vi "TestMirao52e.vi"() -> ()   [LabVIEW 2011]
doc: "This VI is designed to be used with the UDP Receiver VI. Run the UDP Receiver.vi first.\n\nThe UDP protocol differs from TCP in that there is no error-checking with the packets of information that are sent, and thus no guarantee whatsoever that an intended recipient will actually receive a given piece of data.\n\nUDP does offer the ability to \"broadcast\" data across a network--simply specify an IP Address of all ones (255.255.255.255) to attempt to broadcast information network-wide. Keep in mind that routers and other network hardware will generally refuse to forward the broadcast beyond certain points, so the extent of the broadcast will in practice be limited."
panel:
  out "Success":bool
  out "last number of received shapes":u64
  out "sending port":u16
  in  "Remote Host":string="localhost"
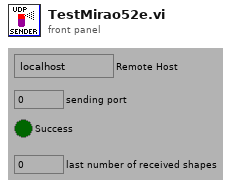
[diagram p1: front panel]
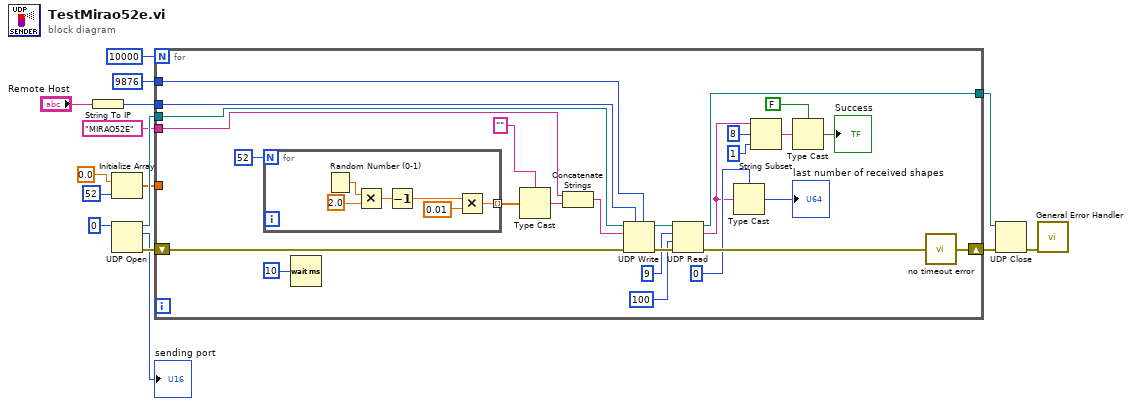
[diagram p0: block diagram]
diagram:
  n1 = String To IP(1:"Remote Host") -> (0:w8:u32)
  n2 = Initialize Array(0.0 ("element"), 52 ("dimension size")) -> (w5:dbl[])
  n3 = UDP Open(11:u16 0 ("port")) -> (port=w15:refnum<k16>, 0:w13:errorcluster, 2:→"sending port":u16)  [unwired: 1 in, 3 out]
  n4 = for {
    N: u32 10000 ("Remote Port") -> [_]
    tunnel: w15 -> [w39]
    tunnel: w8 -> [w41]
    tunnel: u16 9876 ("Remote Port") -> [w40]
    shift-right: [w25] -> w12
    shift-left: w13 -> [w38]
    tunnel: [w29] -> w11
    tunnel: w5 -> [_]
    tunnel: "MIRAO52E" ("data out") -> [w27]
    n5 = for {
      N: 52 -> [_]
      tunnel: [w45] -> w36 mode=indexing
      n6 = Random Number (0-1)() -> (number: 0 to 1=w47:dbl)
      n7 = Multiply(x=w47, y=2.0) -> (x*y=w43:dbl)
      n8 = Decrement(x=w43) -> (x-1=w42:dbl)
      n9 = Multiply(x=w42, y=0.01) -> (x*y=w45:dbl)
    }
    n10 = Wait (ms)(milliseconds to wait=u32 10 ("millisecond multiple")) -> ()  [unwired: 1 out]
    n11 = Type Cast(type="", x=w36) -> (*(type *) &x=w33:string)
    n12 = Concatenate Strings(w27, w33) -> (w34:string)
    n13 = UDP Write(address=w41, port or service name=w40, connection ID=w39, data in=w34, 8:w38) -> (error out=w30:errorcluster, 3:w31:refnum<k16>)  [unwired: 1 out]
    n14 = UDP Read(connection ID=w31, max size (548)=9, timeout ms (25000)=100, 8:w30) -> (data out=w22:string, error out=w26:errorcluster, 3:w29:refnum<k16>)  [unwired: 2 out]
    n15 = Type Cast(type=u64 0 ("Port"), x=w22) -> (*(type *) &x=→"last number of received shapes":u64)
    n16 = String Subset(string=w22, offset (0)=8, length (rest)=1 ("length (rest)")) -> (substring=w19:string)
    n17 = Type Cast(type=FALSE ("Success"), x=w19) -> (*(type *) &x=→"Success":bool)
    n18 = call "no timeout error.vi"("error in (no error)"=w26) -> ("error out"=w25:errorcluster)
  }
  n19 = UDP Close(connection ID=w11, 8:w12) -> (error out=w10:errorcluster)  [unwired: 1 out]
  n20 = call <vilib>:"General Error Handler.vi"("error in (no error)"=w10) -> ()  [unwired: 1 in, 14 out]
